vi "(SubVI)_CLosedLoop16_Processing_loop2.vi"(0 "Index of for loop":i32, 1 "element":T1, 2 "Doppler 2D":bool=TRUE, 3 "velocity_profile 3":dbl[][](array[numeric]), 4 "Image Avg":dbl=1.0 min=1.0 max=100.0 step=1.0, 5 "first row":dbl[](array[numeric]), 6 "output cluster":T2, 7 "Power 2D":dbl=0.2 min=0.01 max=0.9 step=0.01, 8 "Num of cross-section per image":i32, 9 "Period":dbl, 11 "ROI":cluster{"ROI_Bot":i32, "ROI_Top":i32}, 13 "Direct Dpp":bool=TRUE, 15 "# Cores":i32=4, 17 "Array":dbl[][](array[numeric]), 19 "Stop Button":bool) -> (14 "Depth profile 2":dbl[][](array[numeric]), 20 "FFT":dbl[](array[numeric]), 21 "velocity_profile shift register":dbl[][](array[numeric]), 22 "Frm#, SmDpp":T3, 23 "Doppler 2D":dbl[][](array[numeric]), 24 "error out 4":errorcluster)   [LabVIEW 2019]
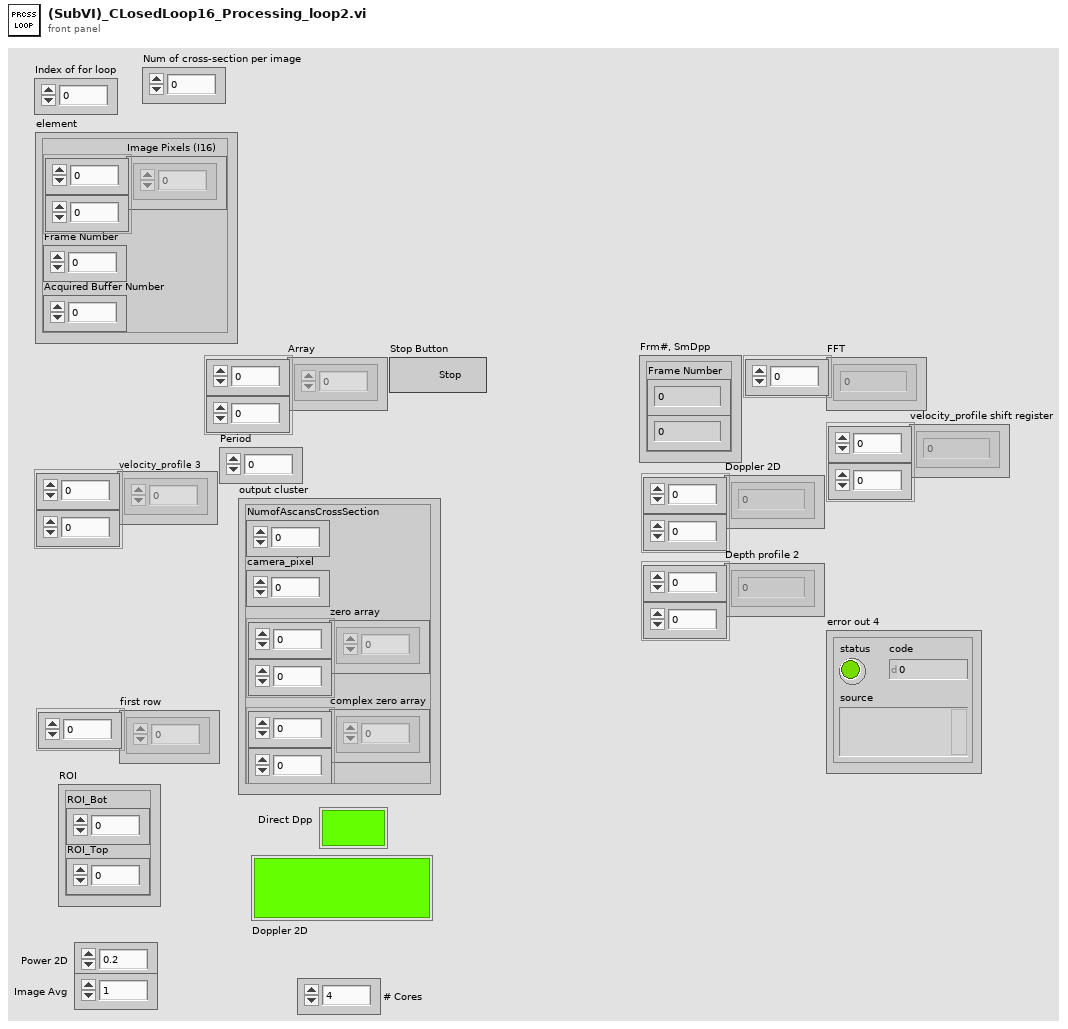
[diagram p1: front panel]
types:
  T1 = cluster{"Image Pixels (I16)":i16[][], "Frame Number":dbl, "Acquired Buffer Number":dbl}
  T2 = cluster{"NumofAscansCrossSection":i32, "camera_pixel":i32, "zero array":dbl[][], "complex zero array":dbl[][]}
  T3 = cluster{"Frame Number":dbl, "Numeric Control":dbl}
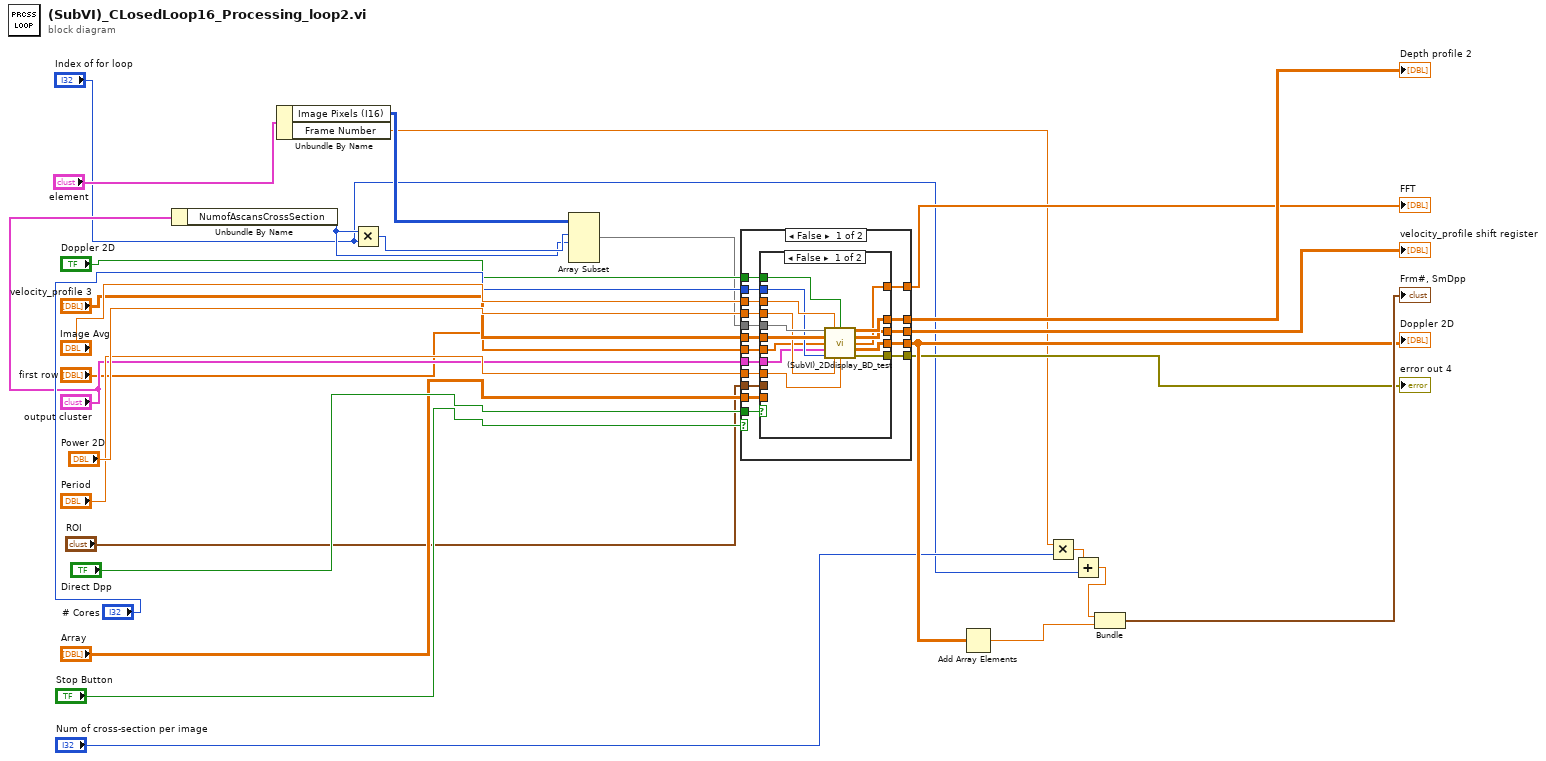
[diagram p0: block diagram]
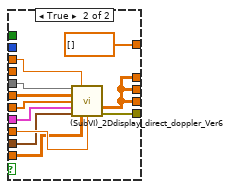
[diagram p2: hidden frame]
diagram:
  n1 = Unbundle By Name("output cluster") -> ("NumofAscansCrossSection"=w6:i32)
  n2 = Unbundle By Name("element") -> ("Image Pixels (I16)"=w26:i16[][], "Frame Number"=w5:dbl)
  n3 = Multiply(x=w6, y="Index of for loop") -> (x*y=w7:i32)
  n4 = Array Subset(array=w26, index (row)=w7, length (row)=w6) -> (w11:i16[][])  [unwired: 2 in]
  n5 = case shown="False" "Stop Button" {
    tunnel: "first row" -> [w46 _]
    tunnel: "output cluster" -> [w41 _]
    tunnel: "velocity_profile 3" -> [w45 w73]
    tunnel: [w44 _] -> w14
    tunnel: [w43 w73] -> w8
    tunnel: "Period" -> [w42 _]
    tunnel: [w40 w72] -> w20
    tunnel: "Doppler 2D" -> [w39 _]
    tunnel: "Image Avg" -> [w38 _]
    tunnel: [w37 _] -> w24
    tunnel: "Power 2D" -> [w36 _]
    tunnel: "Direct Dpp" -> [w35 _]
    tunnel: [w34 _] -> w23
    tunnel: w11 -> [w33 _]
    tunnel: "ROI" -> [w32 _]
    tunnel: "# Cores" -> [w31 _]
    tunnel: "Array" -> [w30 w72]
    frame False {
      n6 = case shown="False" w35 {
        tunnel: w46 -> [w47 w61]
        tunnel: w45 -> [w59 w71]
        tunnel: [w50 w69] -> w44
        tunnel: [w53 w68] -> w43
        tunnel: w42 -> [w57 w70]
        tunnel: w41 -> [w48 w64]
        tunnel: [w51 w68] -> w40
        tunnel: w39 -> [w55 _]
        tunnel: w38 -> [w56 w63]
        tunnel: [w54 w68] -> w37
        tunnel: w36 -> [w58 _]
        tunnel: [w52 dbl[] [] ("Image 2")] -> w34
        tunnel: w33 -> [w60 w65]
        tunnel: w32 -> [_ w66]
        tunnel: w31 -> [w49 _]
        tunnel: w30 -> [_ w62]
        frame False {
          n7 = call "(SubVI)_2Ddisplay_BD_test.vi"("data"=w60, "Image Avg 2D"=w56, "Doppler 2D"=w55, "zero array"=w59, "first row"=w47, "input cluster 3"=w48, "# of Cores"=w49, "Power 2D"=w58, "Period"=w57) -> ("Image"=w54:dbl[][], "buffer out"=w53:dbl[][], "Image 2"=w52:dbl[], "velocity_profile"=w51:dbl[][], "error out"=w50:errorcluster)  [unwired: 2 in]
        }
        frame True {
          n8 = call "(SubVI)_2Ddisplay_direct_doppler_Ver6.vi"("Data"=w65, "Image Avg 2D"=w63, "zero array"=w71, "first row"=w61, "input cluster 3"=w64, "ROI"=w66, "VelcityProfile"=w62, "Numeric"=w70) -> ("velocity_profile"=w68:dbl[][], "error out 4"=w69:errorcluster)  [unwired: 5 in, 1 out]
        }
      }
    }
    frame True {
    }
  }
  "Doppler 2D" <- w20
  "FFT" <- w23
  "Depth profile 2" <- w24
  "velocity_profile shift register" <- w8
  "error out 4" <- w14
  n9 = Add Array Elements(numeric array=w20) -> (sum=w12:dbl)
  n10 = Multiply(x=w5, y="Num of cross-section per image") -> (x*y=w3:dbl)
  n11 = Add(x=w3, y="Index of for loop") -> (x+y=w1:dbl)
  n12 = Bundle(w1, "element"=w12) -> (→"Frm#, SmDpp":cluster{dbl, "element":dbl})  [unwired: 1 in]
